vi "Open Pipe.vi"   [LabVIEW 2013, in "Pipes.lvlib"]
uses:
  Pipes.lvlib
  Classes/Unix Pipe Writer/Unix Pipe Writer.lvclass
  Classes/Unix Pipe Reader/Unix Pipe Reader.lvclass
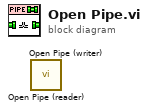
[diagram p0: block diagram]
diagram:
  n1 = call "Open Pipe (reader).vi"() -> ()  [unwired: 10 in, 2 out]
  n2 = call "Open Pipe (writer).vi"() -> ()  [unwired: 10 in, 2 out]
